vi "Read Measurement (N Cycle Jitter).vi"(0 "VISA resource name":refnum<visa-resource-name>, 1 "Number Cycle (5)":i32=5 format="%.0g", 2 "Start Cycle (1)":i32=1 format="%.0g", 5 "Measurement Source (1: Channel 1)":i32(ring)=1 caption="Channel (1: Channel 1)" items=["Channel 1"=1, "Channel 2"=2, "Channel 3"=3, "Channel 4"=4, "Function 1"=5, "Function 2"=6, "Function 3"=7, "Function 4"=8, "Memory 1"=9, "Memory 2"=10, "Memory 3"=11, "Memory 4"=12, "Clock"=15, "MTrend"=16, "MSpectrum"=17, "Equalized"=18, "DIG 0"=20, "DIG 1"=21, "DIG 2"=22, "DIG 3"=23, "DIG 4"=24, "DIG 5"=25, "DIG 6"=26, "DIG 7"=27, "DIG 8"=28, "DIG 9"=29, "DIG 10"=30, "DIG 11"=31, "DIG 12"=32, "DIG 13"=33, "DIG 14"=34, "DIG 15"=35], 7 "Edge (0: Rising)":i32(ring) items=["Rising", "Falling"], 9 "Maximum Time (10000ms)":u32=10000, 11 "error in (no error)":errorcluster) -> (4 "VISA resource name out":refnum<visa-resource-name>, 6 "N Cycle Jitter (s)":dbl caption="N cycle jitter (s)", 15 "error out":errorcluster)   [LabVIEW 2020, in "Agilent 90000 Series.lvlib"]
doc: "Measures the N cycle jitter of the waveform. \n\nThis VI initiates an acquisition on the channel that the end-user defines. It then waits for the acquisition to complete, obtains a waveform measurement on the channel the end-user specifies, and returns the measurement value."
uses:
  Agilent 90000 Series.lvlib
  Low Level/Fetch Measurement (N Cycle Jitter).vi
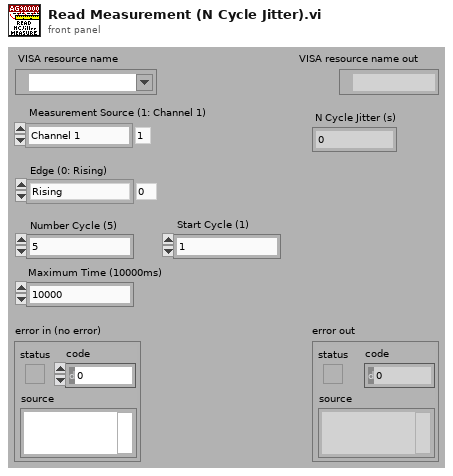
[diagram p1: front panel]
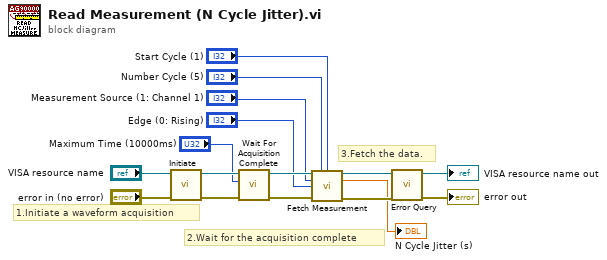
[diagram p0: block diagram]
diagram:
  # "3.Fetch the data."
  # "2.Wait for the acquisition complete"
  # "1.Initiate a waveform acquisition"
  n1 = call "Initiate.vi"("error in (no error)"="error in (no error)", "VISA resource name"="VISA resource name") -> ("error out"=w14:errorcluster, "VISA resource name out"=w13:refnum<visa-resource-name>)  [unwired: 8 out]
  n2 = call "Wait For Acquisition Complete.vi"("error in (no error)"=w14, "Maximum Time (10000ms)"="Maximum Time (10000ms)", "VISA resource name"=w13) -> ("error out"=w11:errorcluster, "VISA resource name out"=w12:refnum<visa-resource-name>)  [unwired: 7 out]
  n3 = call-poly "Fetch Measurement.vi"("VISA resource name"=w12, "Number Cycle (5)"="Number Cycle (5)", "Start Cycle (1)"="Start Cycle (1)", "Measurement Source (1: Channel 1)"="Measurement Source (1: Channel 1)", "Edge (0: Rising)"="Edge (0: Rising)", "error in (no error)"=w11) -> ("VISA resource name out"=w10:refnum<visa-resource-name>, "N Cycle Jitter (s)"=→"N Cycle Jitter (s)":dbl, "error out"=w9:errorcluster)  [unwired: 1 in, 6 out]
  n4 = call "Error Query.vi"("error in (no error)"=w9, "VISA resource name"=w10) -> ("error out"=→"error out":errorcluster, "VISA resource name out"=→"VISA resource name out":refnum<visa-resource-name>)  [unwired: 8 out]
